vi "Configure ALC.vi"(0 "VISA resource name":refnum<visa-resource-name>, 1 "Enable ALC (T:Enable)":bool=TRUE, 5 "ALC Level (1 dB)":dbl=1.0, 7 "Enable Automatic Bandwidth (T:Enable)":bool=TRUE, 9 "ALC Bandwidth (0: 100 Hz)":u16(ring) items=["100 Hz", "1 kHz", "10 kHz", "100 kHz"], 11 "error in (no error)":errorcluster, 12 "ALC Source (0: Internal)":u16(ring) items=["Internal", "External Detector", "Millimeter-wave"], 13 "External Detector Coupling Factor (16 dB)":dbl=16.0) -> (4 "VISA resource name out":refnum<visa-resource-name>, 15 "error out":errorcluster)   [LabVIEW 2011, in "Agilent PSG MXG Series.lvlib"]
doc: "Configures ALC (automatic leveling control) state, ALC level, ALC bandwidth, and ALC source of the signal generator."
uses:
  Agilent PSG MXG Series.lvlib
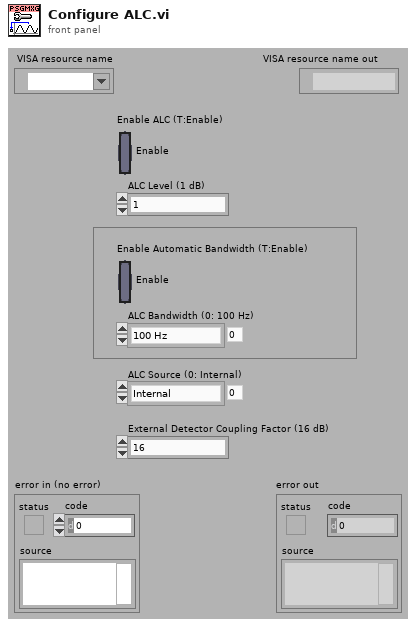
[diagram p1: front panel]
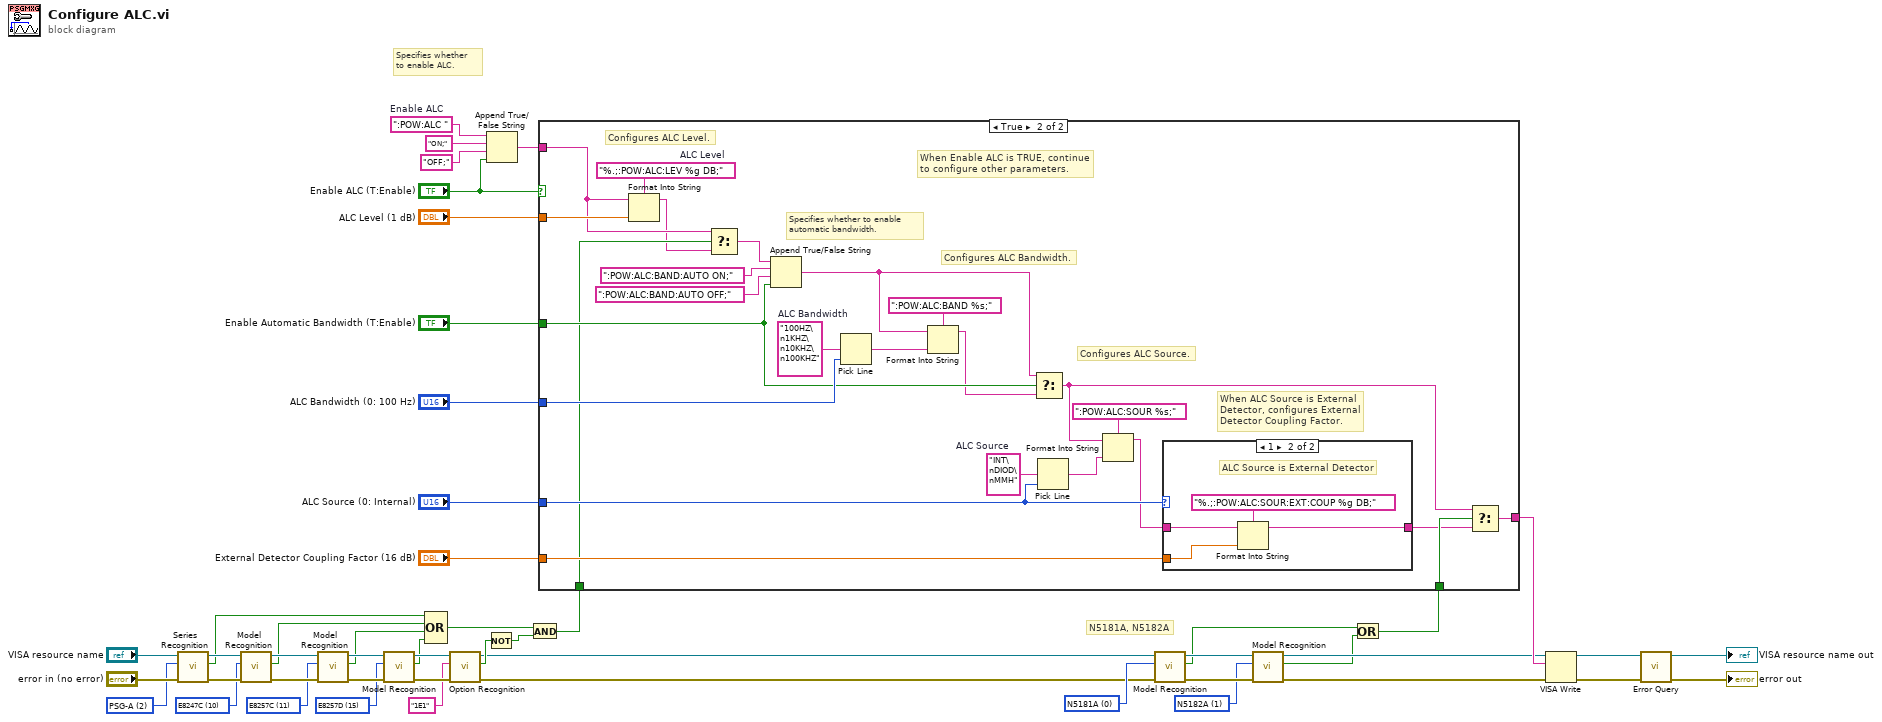
[diagram p0: block diagram]
diagram:
  w14 = u16 15 items=["N5181A"=0, "N5182A"=1, "N5183A"=2, "E8241A"=5, "E8244A"=6, "E8251A"=7, "E8254A"=8, "E8247C"=10, "E8257C"=11, "E8267C"=12, "E8257D"=15, "E8267D"=16] ("Model Type (0: N5181A)")
  w17 = u16 11 items=["N5181A"=0, "N5182A"=1, "N5183A"=2, "E8241A"=5, "E8244A"=6, "E8251A"=7, "E8254A"=8, "E8247C"=10, "E8257C"=11, "E8267C"=12, "E8257D"=15, "E8267D"=16] ("Model Type (0: N5181A)")
  w20 = u16 10 items=["N5181A"=0, "N5182A"=1, "N5183A"=2, "E8241A"=5, "E8244A"=6, "E8251A"=7, "E8254A"=8, "E8247C"=10, "E8257C"=11, "E8267C"=12, "E8257D"=15, "E8267D"=16] ("Model Type (0: N5181A)")
  w23 = u16 2 items=["MXG", "PSG", "PSG-A", "PSG-C", "PSG-D"] ("Series Type (0: MXG)")
  w29 = u16 1 items=["N5181A"=0, "N5182A"=1, "N5183A"=2, "E8241A"=5, "E8244A"=6, "E8251A"=7, "E8254A"=8, "E8247C"=10, "E8257C"=11, "E8267C"=12, "E8257D"=15, "E8267D"=16] ("Model Type (0: N5181A)")
  w34 = u16 0 items=["N5181A"=0, "N5182A"=1, "N5183A"=2, "E8241A"=5, "E8244A"=6, "E8251A"=7, "E8254A"=8, "E8247C"=10, "E8257C"=11, "E8267C"=12, "E8257D"=15, "E8267D"=16] ("Model Type (0: N5181A)")
  w49 = ":POW:ALC "  # Enable ALC
  # "N5181A, N5182A"
  # "Specifies whether\nto enable ALC."
  n1 = call "Series Recognition.vi"("error in (no error)"="error in (no error)", "Series Type (0: MXG)"=w23, "VISA resource name"="VISA resource name") -> ("error out"=w21:errorcluster, "Is Series Correct"=w10:bool, "VISA resource name out"=w22:refnum<visa-resource-name>)  [unwired: 6 in]
  n2 = call "Model Recognition.vi"("error in (no error)"=w21, "Model Type (0: N5181A)"=w20, "VISA resource name"=w22) -> ("error out"=w18:errorcluster, "Is Model Correct"=w9:bool, "VISA resource name out"=w19:refnum<visa-resource-name>)  [unwired: 6 in]
  n3 = call "Model Recognition.vi"("error in (no error)"=w18, "Model Type (0: N5181A)"=w17, "VISA resource name"=w19) -> ("error out"=w15:errorcluster, "Is Model Correct"=w8:bool, "VISA resource name out"=w16:refnum<visa-resource-name>)  [unwired: 6 in]
  n4 = call "Model Recognition.vi"("error in (no error)"=w15, "Model Type (0: N5181A)"=w14, "VISA resource name"=w16) -> ("error out"=w12:errorcluster, "Is Model Correct"=w7:bool, "VISA resource name out"=w13:refnum<visa-resource-name>)  [unwired: 6 in]
  n5 = Compound Arithmetic op=OR(w10, w9, w8, w7) -> (w5:bool)
  n6 = call "Option Recognition.vi"("error in (no error)"=w12, "Option (\"\")"="1E1" ("Option (\"\")"), "VISA resource name"=w13) -> ("error out"=w1:errorcluster, "Is Option Installed"=w6:bool, "VISA resource name out"=w2:refnum<visa-resource-name>)  [unwired: 6 in]
  n7 = Not(x=w6) -> (.not. x?=w4:bool)
  n8 = Append True/False String(1:"Enable ALC (T:Enable)", 2:"OFF;" ("false string"), 3:"ON;" ("true string"), 4:w49) -> (0:w47:string)
  n9 = And(x=w5, y=w4) -> (x .and. y?=w3:bool)
  n10 = call "Model Recognition.vi"("error in (no error)"=w1, "Model Type (0: N5181A)"=w34, "VISA resource name"=w2) -> ("error out"=w32:errorcluster, "Is Model Correct"=w27:bool, "VISA resource name out"=w33:refnum<visa-resource-name>)  [unwired: 6 in]
  n11 = call "Model Recognition.vi"("error in (no error)"=w32, "Model Type (0: N5181A)"=w29, "VISA resource name"=w33) -> ("error out"=w30:errorcluster, "Is Model Correct"=w28:bool, "VISA resource name out"=w31:refnum<visa-resource-name>)  [unwired: 6 in]
  n12 = Or(x=w27, y=w28) -> (x .or. y?=w26:bool)
  n13 = case shown="True" "Enable ALC (T:Enable)" {
    tunnel: w47 -> [w50 w53]
    tunnel: "ALC Level (1 dB)" -> [_ w75]
    tunnel: "ALC Bandwidth (0: 100 Hz)" -> [_ w70]
    tunnel: "Enable Automatic Bandwidth (T:Enable)" -> [_ w68]
    tunnel: "ALC Source (0: Internal)" -> [_ w58]
    tunnel: "External Detector Coupling Factor (16 dB)" -> [_ w59]
    tunnel: [w50 w62] -> w40
    tunnel: w26 -> [_ w60]
    tunnel: w3 -> [_ w54]
    frame False {
      # "When Enable ALC\nis FALSE, do nothing."
    }
    frame True {
      w63 = "INT\nDIOD\nMMH"  # ALC Source
      w71 = "100HZ\n1KHZ\n10KHZ\n100KHZ"  # ALC Bandwidth
      w74 = "%.;:POW:ALC:LEV %g DB;"  # ALC Level
      # "When ALC Source is External\nDetector, configures External\nDetector Coupling Factor."
      # "Configures ALC Source."
      # "Configures ALC Bandwidth."
      # "Specifies whether to enable\nautomatic bandwidth."
      # "Configures ALC Level."
      # "When Enable ALC is TRUE, continue\nto configure other parameters."
      n14 = Format Into String(format string=w74, initial string=w53, w75) -> (resulting string=w52:string)  [unwired: 1 in, 1 out]
      n15 = Select(t=w53, s=w54, f=w52) -> (s? t:f=w51:string)
      n16 = Append True/False String(1:w68, 2:":POW:ALC:BAND:AUTO OFF;" ("format string"), 3:":POW:ALC:BAND:AUTO ON;" ("format string"), 4:w51) -> (0:w67:string)
      n17 = Pick Line(multi-line string=w71, line index=w70) -> (output string=w69:string)  [unwired: 1 in]
      n18 = Format Into String(format string=":POW:ALC:BAND %s;", initial string=w67, w69) -> (resulting string=w66:string)  [unwired: 1 in, 1 out]
      n19 = Select(t=w67, s=w68, f=w66) -> (s? t:f=w61:string)
      n20 = Pick Line(multi-line string=w63, line index=w58) -> (output string=w64:string)  [unwired: 1 in]
      n21 = Format Into String(format string=":POW:ALC:SOUR %s;", initial string=w61, w64) -> (resulting string=w56:string)  [unwired: 1 in, 1 out]
      n22 = case shown="1" w58 {
        tunnel: w59 -> [_ w79]
        tunnel: [w76 w78] -> w57
        tunnel: w56 -> [w76 w77]
        frame 0, Default {
          # "ALC Source is Internal or\nMillimeter-wave"
        }
        frame 1 {
          # "ALC Source is External Detector"
          n23 = Format Into String(format string="%.;:POW:ALC:SOUR:EXT:COUP %g DB;", initial string=w77, w79) -> (resulting string=w78:string)  [unwired: 1 in, 1 out]
        }
      }
      n24 = Select(t=w61, s=w60, f=w57) -> (s? t:f=w62:string)
    }
  }
  n25 = VISA Write(VISA resource name=w31, write buffer=w40, error in (no error)=w30) -> (VISA resource name out=w39:refnum<visa-resource-name>, error out=w38:errorcluster)  [unwired: 1 out]
  n26 = call "Error Query.vi"("error in (no error)"=w38, "VISA resource name"=w39) -> ("error out"=→"error out":errorcluster, "VISA resource name out"=→"VISA resource name out":refnum<visa-resource-name>)  [unwired: 6 in, 2 out]
